vi "error_w_context.vi"(8 "error in (no error)":errorcluster, 11 "error source":string) -> ()   [LabVIEW 2012]
uses:
  <vilib>/Utility/error.llb/DialogType.ctl
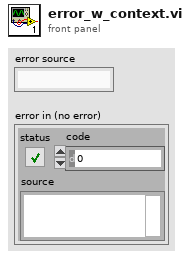
[diagram p1: front panel]
types:
  T1 = typedef "DialogType.ctl" = u16
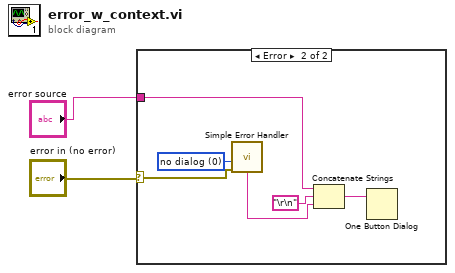
[diagram p0: block diagram]
diagram:
  n1 = case shown="Error" "error in (no error)" {
    selector: "error in (no error)" -> [_ w8]
    tunnel: "error source" -> [_ w6]
    frame No Error {
    }
    frame Error {
      w7 = T1 0 items=["no dialog", "OK message", "continue or stop message", "OK message + warnings", "continue/stop + warnings"] ("type of dialog (OK msg:1)")
      n2 = call <vilib>:"Simple Error Handler.vi"("type of dialog (OK msg:1)"=w7, "error in (no error)"=w8) -> ("message"=w4:string)  [unwired: 3 in, 4 out]
      n3 = Concatenate Strings(w6, "\r\n", w4) -> (w3:string)
      n4 = One Button Dialog(message=w3) -> ()  [unwired: 1 in, 1 out]
    }
  }
